vi "GetLocalComputerName.vi"(8 "error in (no error)":errorcluster) -> (0 "error out":errorcluster, 1 "Full Name":string, 2 "Name":string)   [LabVIEW 2013]
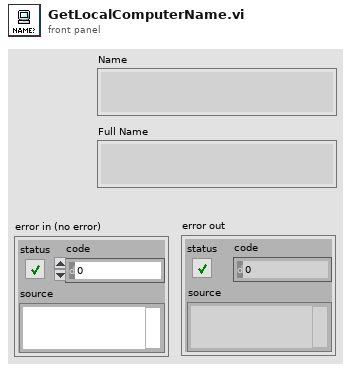
[diagram p1: front panel]
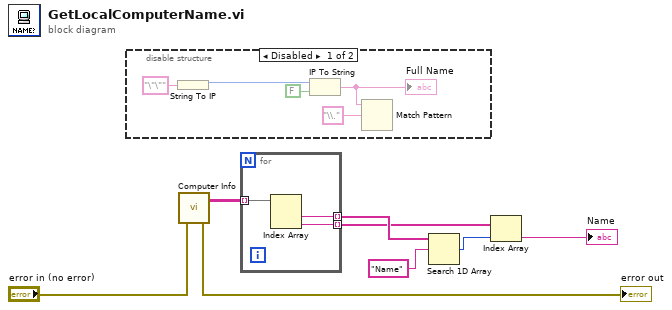
[diagram p0: block diagram]
diagram:
  n1 = disable-structure shown="Disabled" {
    frame Disabled {
      n2 = String To IP(1:"\"\"" ("name")) -> (0:w12:u32)
      n3 = IP To String(1:FALSE ("dot notation? (F)"), 2:w12) -> (0:w9:string)
      "Full Name" <- w9
      n4 = Match Pattern(string=w9, regular expression="\\.") -> ()  [unwired: 1 in, 4 out]
    }
    frame Enabled {
    }
  }
  n5 = call "Computer Info.vi"("error in (no error)"="error in (no error)") -> ("error out"=→"error out":errorcluster, "Computer Info"=w8:string[][])  [unwired: 1 in]
  n6 = for {
    tunnel: w8 -> [w16] mode=indexing
    tunnel: [w15] -> w5 mode=indexing
    tunnel: [w14] -> w4 mode=indexing
    n7 = Index Array(array=w16) -> (element #1=w15:string, element #2=w14:string)  [unwired: 2 in]
  }
  n8 = Search 1D Array(1D array=w5, element="Name") -> (index of element=w6:i32)  [unwired: 1 in]
  n9 = Index Array(array=w4, index=w6) -> (element=→"Name":string)
